vi "Process Keystroke.vi"(0 "Listbox":refnum<vi>, 1 "Default":string[](array[string]), 2 "can move":bool, 5 "ScanCode":i16, 7 "Row":i32, 9 "Properties":T3, 11 "error in (no error)":errorcluster, 12 "Columns":T1[](array[typedef])) -> (6 "Event type":T4, 8 "Row Out":i32, 10 "data changed?":bool, 15 "error out":errorcluster)   [LabVIEW 2020, in "KTable.xctl"]
uses:
  KTable.xctl
  Event Type.ctl
  Table Properties.ctl
  ColumnSpec.ctl
  ColumnType.ctl
  Array Manipulation VIs/Array-Dimensions (2D string).vi
panel:
  out "Listbox Out":refnum<vi>
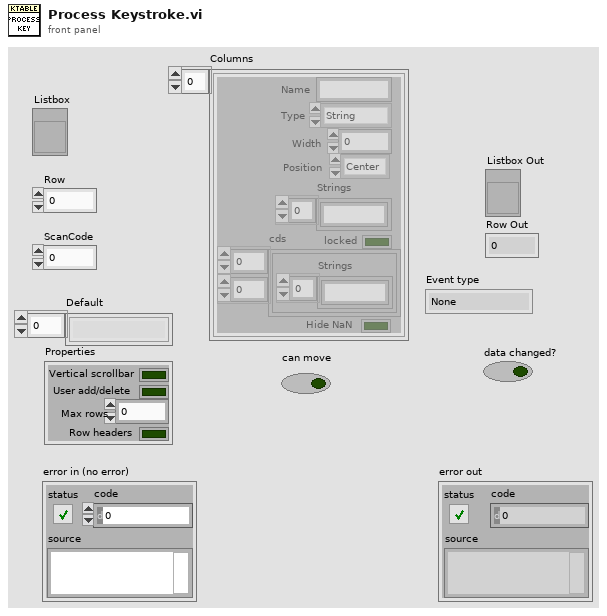
[diagram p1: front panel]
types:
  T1 = typedef "KTable.xctl/ColumnSpec.ctl" = cluster{"Name":string, "Type":T2, "Width":i32, "Strings":string[], "Position":enum16{"Left", "Center", "Right"}, "locked":bool, "cds":cluster{"Strings":string[]}[][], "Hide NaN":bool}
  T2 = typedef "KTable.xctl/ColumnType.ctl" = enum16{"String", "Enum", "Int", "Double", "Boolean", "Ring", "Formula", "Color"}
  T3 = typedef "KTable.xctl/Table Properties.ctl" = cluster{"Vertical scrollbar":bool, "User add/delete":bool, "Max rows":i32, "Row headers":bool}
  T4 = typedef "KTable.xctl/Event Type.ctl" = enum16{"None", "Selection", "Edit", "Insert", "Delete", "Up", "Down", "Duplicate"}
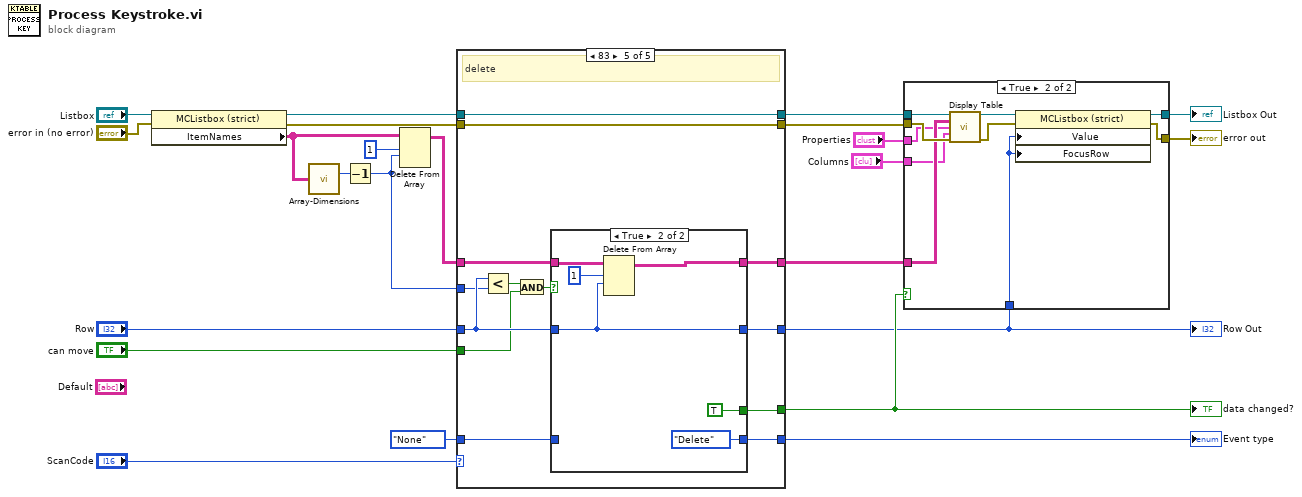
[diagram p0: block diagram]
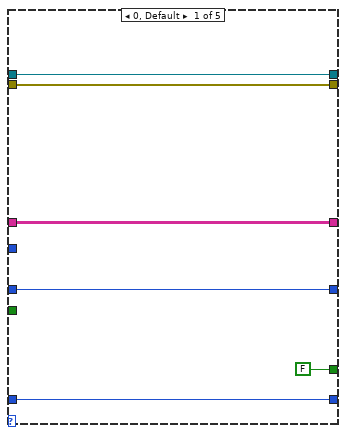
[diagram p2: hidden frame]
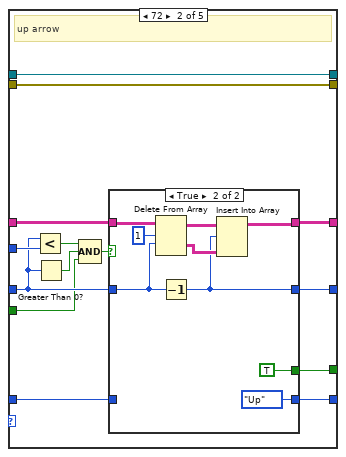
[diagram p3: hidden frame]
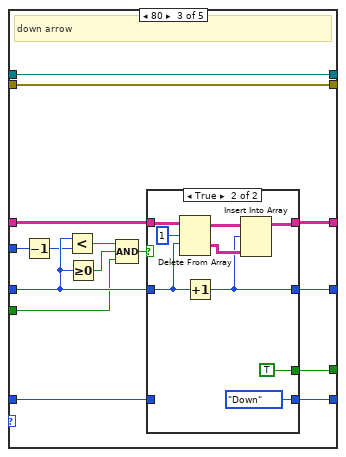
[diagram p5: hidden frame]
diagram:
  n1 = property class="MCListbox (strict)"(reference="Listbox", error in="error in (no error)") -> (reference out=w4:refnum<vi>, error out=w3:errorcluster, "ItemNames"=w13:string[][])
  n2 = call-poly "Array-Dimensions.vi"("2D Array"=w13) -> ("# rows"=w12:i32)  [unwired: 13 in, 1 out]
  n3 = Decrement(x=w12) -> (x-1=w11:i32)
  n4 = Delete From Array(array=w13, length=1, index (row)=w11) -> (array with subset deleted=w15:string[][])  [unwired: 1 in, 1 out]
  n5 = case shown="83" "ScanCode" {
    tunnel: [FALSE w39 w66 _ w95] -> w19
    tunnel: "Row" -> [w28 w36 w63 w86 w98]
    tunnel: w15 -> [w27 w43 w70 w87 w100]
    tunnel: w11 -> [_ w38 w65 _ w94]
    tunnel: [w28 w41 w68 w86 w97] -> w10
    tunnel: [w27 w40 w67 w87 w96] -> w16
    tunnel: Event_Type."None" ("Type") -> [w26 w34 w60 w85 w92]
    tunnel: [w26 w33 w59 w85 w93] -> w8
    tunnel: [w25 w32 w58 w84 w91] -> w5
    tunnel: w4 -> [w25 w32 w58 w84 w91]
    tunnel: w3 -> [w24 w31 w57 w83 w90]
    tunnel: [w24 w31 w57 w83 w90] -> w2
    tunnel: "can move" -> [_ w30 w56 _ w88]
    frame 0, Default {
    }
    frame 72 {
      # "up arrow"
      n6 = Less?(x=w36, y=w38) -> (x < y?=w42:bool)
      n7 = Greater Than 0?(x=w36) -> (x > 0?=w35:bool)
      n8 = Compound Arithmetic op=AND(w42, w35, w30) -> (w37:bool)
      n9 = case shown="True" w37 {
        tunnel: w43 -> [w45 w55]
        tunnel: w36 -> [w46 w53]
        tunnel: [w45 w49] -> w40
        tunnel: [w46 w48] -> w41
        tunnel: [_ TRUE] -> w39
        tunnel: w34 -> [w44 _]
        tunnel: [w44 Event_Type."Up" ("Type")] -> w33
        frame False {
        }
        frame True {
          n10 = Delete From Array(array=w55, length=1, index (row)=w53) -> (deleted portion=w50:string[][], array with subset deleted=w51:string[][])  [unwired: 1 in]
          n11 = Decrement(x=w53) -> (x-1=w48:i32)
          n12 = Insert Into Array(array=w51, index (row)=w48, new element=w50) -> (w49:string[][])  [unwired: 1 in]
        }
      }
    }
    frame 80 {
      # "down arrow"
      n13 = Decrement(x=w65) -> (x-1=w61:i32)
      n14 = Less?(x=w63, y=w61) -> (x < y?=w69:bool)
      n15 = Greater Or Equal To 0?(x=w63) -> (x >= 0?=w62:bool)
      n16 = Compound Arithmetic op=AND(w69, w62, w56) -> (w64:bool)
      n17 = case shown="True" w64 {
        tunnel: w70 -> [w72 w82]
        tunnel: w63 -> [w73 w80]
        tunnel: [w72 w76] -> w67
        tunnel: [w73 w75] -> w68
        tunnel: [_ TRUE] -> w66
        tunnel: w60 -> [w71 _]
        tunnel: [w71 Event_Type."Down" ("Type")] -> w59
        frame False {
        }
        frame True {
          n18 = Delete From Array(array=w82, length=1, index (row)=w80) -> (deleted portion=w77:string[][], array with subset deleted=w78:string[][])  [unwired: 1 in]
          n19 = Increment(x=w80) -> (x+1=w75:i32)
          n20 = Insert Into Array(array=w78, index (row)=w75, new element=w77) -> (w76:string[][])  [unwired: 1 in]
        }
      }
    }
    frame 82 {
      # "insert"
    }
    frame 83 {
      # "delete"
      n21 = Less?(x=w98, y=w94) -> (x < y?=w99:bool)
      n22 = And(x=w99, y=w88) -> (x .and. y?=w89:bool)
      n23 = case shown="True" w89 {
        tunnel: w100 -> [w102 w109]
        tunnel: w98 -> [w103 w106]
        tunnel: [w102 w107] -> w96
        tunnel: [w103 w106] -> w97
        tunnel: [_ TRUE] -> w95
        tunnel: [w101 Event_Type."Delete" ("Type")] -> w93
        tunnel: w92 -> [w101 _]
        frame False {
        }
        frame True {
          n24 = Delete From Array(array=w109, length=1, index (row)=w106) -> (array with subset deleted=w107:string[][])  [unwired: 1 in, 1 out]
        }
      }
    }
  }
  "data changed?" <- w19
  "Row Out" <- w10
  "Event type" <- w8
  n25 = case shown="True" w19 {
    tunnel: w5 -> [w111 w121]
    tunnel: w2 -> [w110 w120]
    tunnel: [w111 w116] -> w18
    tunnel: [w110 w115] -> w17
    tunnel: w16 -> [_ w119]
    tunnel: w10 -> [_ w114]
    tunnel: "Properties" -> [_ w113]
    tunnel: "Columns" -> [_ w112]
    frame False {
    }
    frame True {
      n26 = call "Display Table.vi"("Listbox"=w121, "Table Items"=w119, "Properties"=w113, "Columns"=w112, "error in (no error)"=w120) -> ("reference out"=w118:refnum<vi>, "error out"=w117:errorcluster)  [unwired: 9 in]
      n27 = property class="MCListbox (strict)"(reference=w118, error in=w117, "Value"=w114, "FocusRow"=w114) -> (reference out=w116:refnum<vi>, error out=w115:errorcluster)
    }
  }
  "error out" <- w17
  "Listbox Out" <- w18
